vi "NewLINE.vi"() -> ()   [LabVIEW 2010]
uses:
  <vilib>/express/express arith-compare/Formula/XNode/ExpressFormulaBlockNode.xnode
panel:
  out "Numeric":u16
  in  "Array":dbl[](array[numeric])=[37.0]
  in  "Current (mA)":dbl
  in  "Motor GPIB":u8=6
  in  "y-dist":i32
  in  "speed":u16
  in  "x-dist":i32
  out "Dummy":string
  in  "Laser GPIB":u8=10 max=100
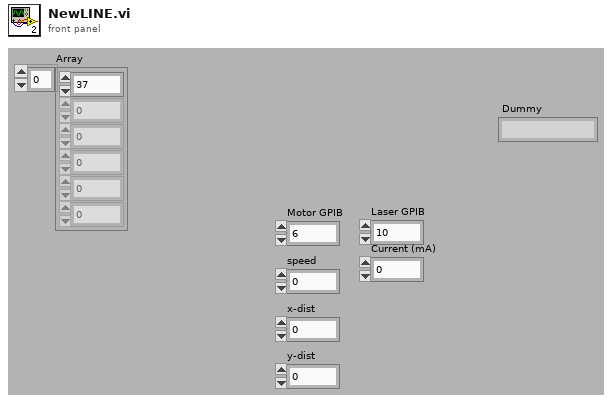
[diagram p1: front panel]
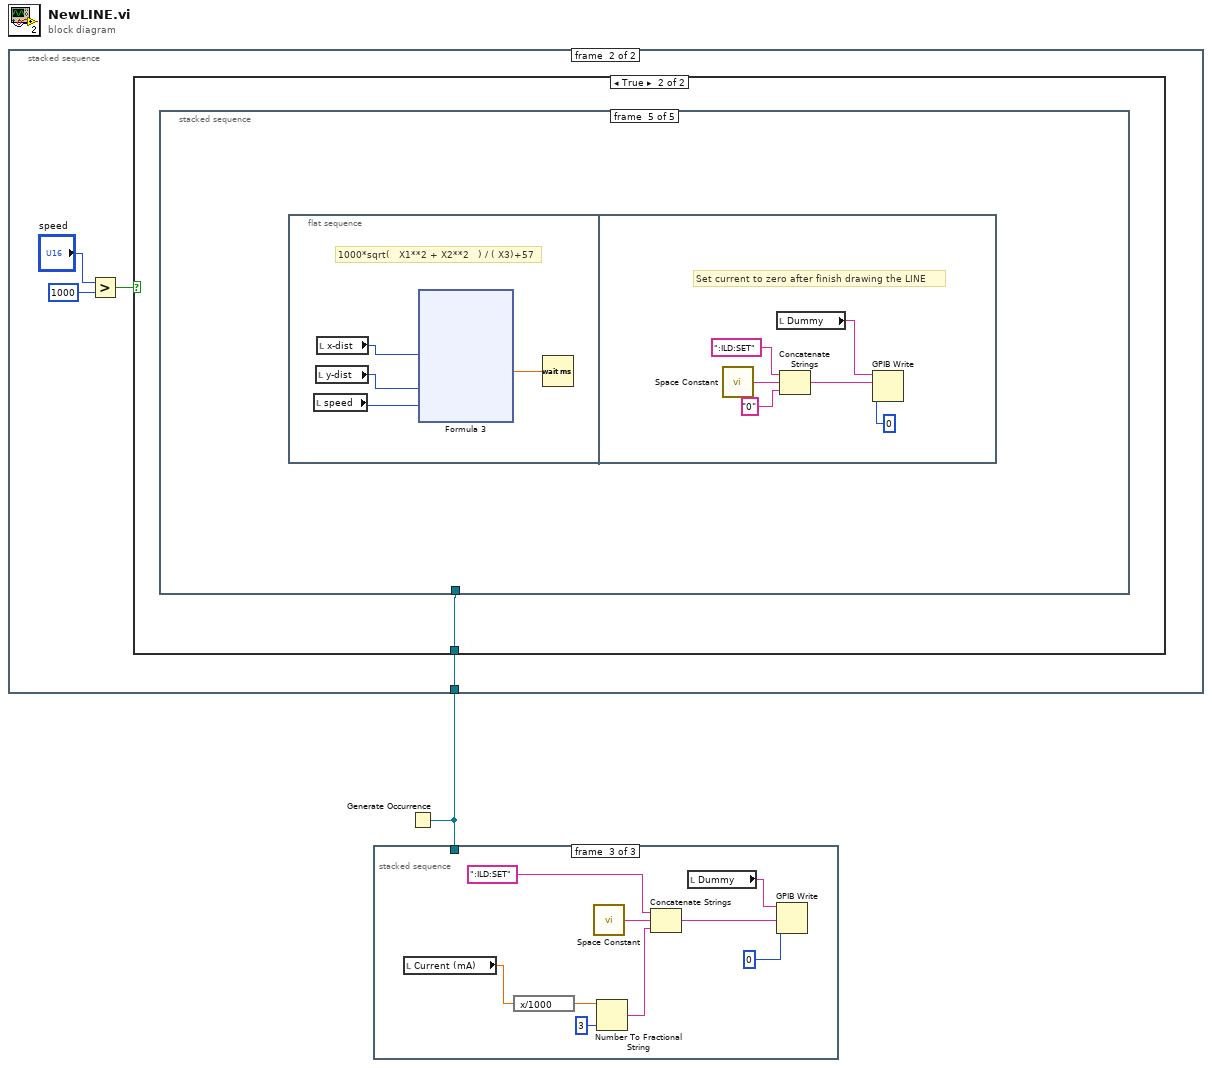
[diagram p0: block diagram]
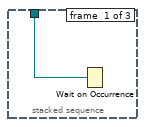
[diagram p2: hidden frame]
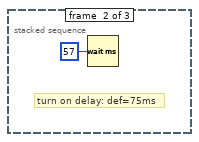
[diagram p3: hidden frame]
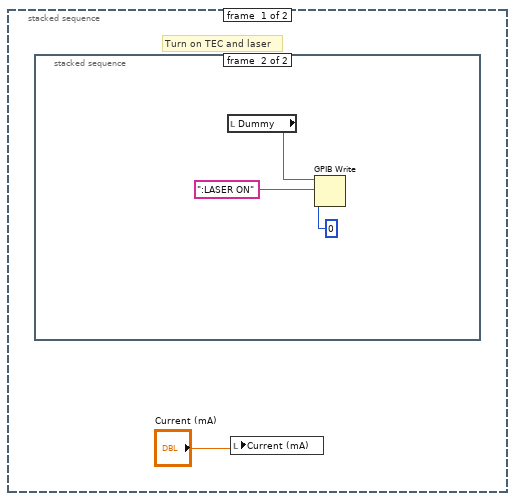
[diagram p4: hidden frame]
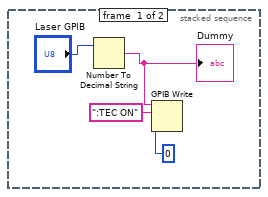
[diagram p5: hidden frame]
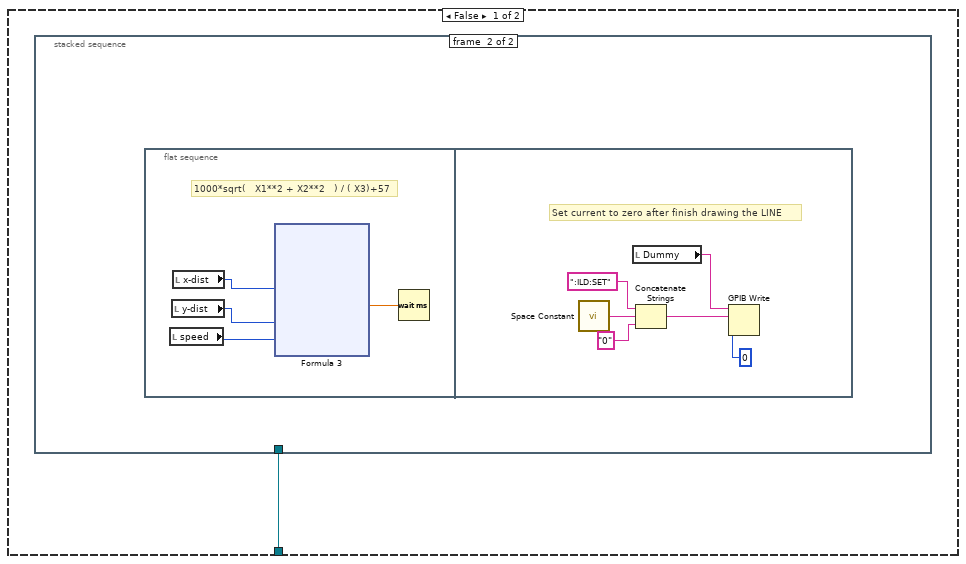
[diagram p6: hidden frame]
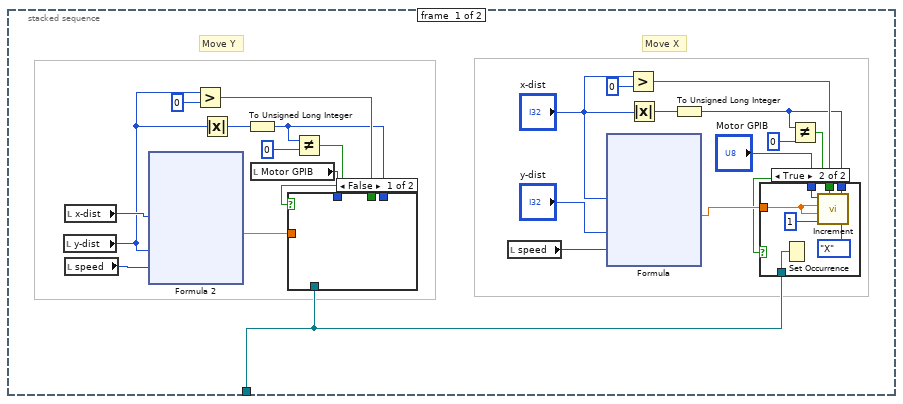
[diagram p7: hidden frame]
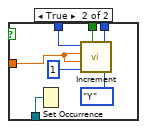
[diagram p9: hidden frame]
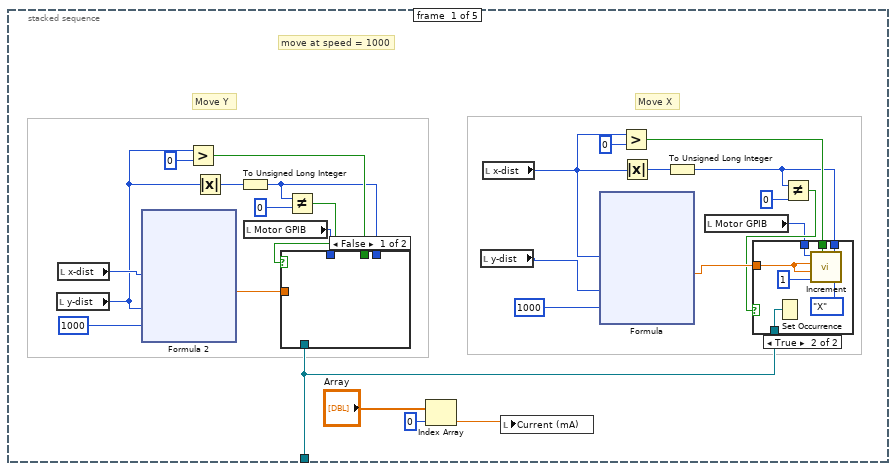
[diagram p10: hidden frame]
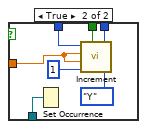
[diagram p12: hidden frame]
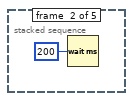
[diagram p13: hidden frame]
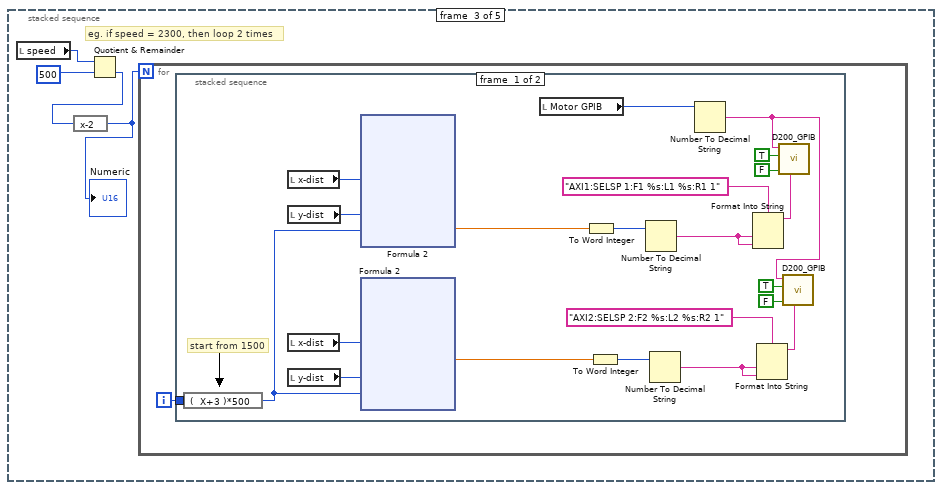
[diagram p14: hidden frame]
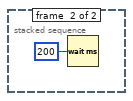
[diagram p15: hidden frame]
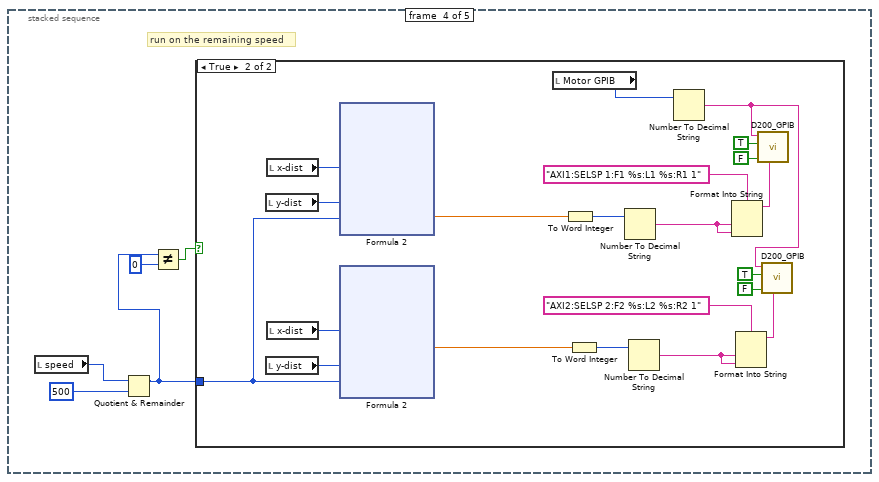
[diagram p16: hidden frame]
diagram:
  n1 = Generate Occurrence() -> (w1:refnum<k4>)
  n2 = stacked-sequence {
    tunnel: w1 -> [_ w11]
    frame #0 {
      # "Turn on TEC and laser"
      n3 = stacked-sequence {
        frame #0 {
          n4 = Number To Decimal String(number="Laser GPIB") -> (decimal integer string=w4:string)  [unwired: 1 in]
          "Dummy" <- w4
          n5 = GPIB Write(0:w4, 1:":TEC ON" ("data"), 2:i16 0 ("mode (0)")) -> ()  [unwired: 2 in, 2 out]
        }
        frame #1 {
          n6 = local read "Dummy"() -> (w8:string)
          n7 = GPIB Write(0:w8, 1:":LASER ON" ("data"), 2:i16 0 ("mode (0)")) -> ()  [unwired: 2 in, 2 out]
        }
      }
      n8 = local write "Current (mA)"("Current (mA)") -> ()
    }
    frame #1 {
      n9 = Greater?(x="speed", y=u16 1000) -> (0:w10:bool)
      n10 = case shown="True" w10 {
        tunnel: w11 -> [w14 w98]
        frame False {
          n11 = stacked-sequence {
            tunnel: w14 -> [w15 _]
            frame #0 {
              # "Move X"
              # "Move Y"
              n12 = local read "y-dist"() -> (w31:i32)
              n13 = local read "x-dist"() -> (w33:i32)
              n14 = local read "speed"() -> (w37:u16)
              n15 = xnode "Formula 2"("X1"=w33, "X2"=w31, "X3"=w37) -> ("Result"=w24:dbl)  [unwired: 1 in, 1 out]
              n16 = Greater?(x=w31, y=0) -> (0:w34:bool)
              n17 = Absolute Value(x=w31) -> (abs(x)=w32:i32)
              n18 = To Unsigned Long Integer(number=w32) -> (unsigned 32bit integer=w22:u32)
              n19 = local read "Motor GPIB"() -> (w36:u8)
              n20 = Not Equal?(x=w22, y=u32 0) -> (x != y?=w20:bool)
              n21 = case shown="False" w20 {
                tunnel: w36 -> [_ w49]
                tunnel: w34 -> [_ w48]
                tunnel: w22 -> [_ w47]
                tunnel: w24 -> [_ w46]
                tunnel: w15 -> [_ w45]
                frame False {
                }
                frame True {
                  n22 = Set Occurrence(w45) -> ()
                  n23 = call "Increment.vi"("GPIB_Addr"=w49, "F Speed"=w46, "L Speed"=w46, "Rate"=u16 1, "CCW 3"=w48, "Distance"=w47, "Axis"=enum16{"X", "Y", "Z", "U", "V", "W"}."Y") -> ()
                }
              }
              n24 = local read "speed"() -> (w16:u16)
              n25 = xnode "Formula"("X1"="x-dist", "X2"="y-dist", "X3"=w16) -> ("Result"=w23:dbl)  [unwired: 1 in, 1 out]
              n26 = Greater?(x="x-dist", y=0) -> (0:w28:bool)
              n27 = Absolute Value(x="x-dist") -> (abs(x)=w25:i32)
              n28 = To Unsigned Long Integer(number=w25) -> (unsigned 32bit integer=w19:u32)
              n29 = Not Equal?(x=w19, y=u32 0) -> (x != y?=w17:bool)
              n30 = case shown="True" w17 {
                tunnel: "Motor GPIB" -> [_ w44]
                tunnel: w28 -> [_ w41]
                tunnel: w19 -> [_ w40]
                tunnel: w23 -> [_ w39]
                tunnel: w15 -> [_ w38]
                frame False {
                }
                frame True {
                  n31 = Set Occurrence(w38) -> ()
                  n32 = call "Increment.vi"("GPIB_Addr"=w44, "F Speed"=w39, "L Speed"=w39, "Rate"=u16 1, "CCW 3"=w41, "Distance"=w40, "Axis"=enum16{"X", "Y", "Z", "U", "V", "W"}."X") -> ()
                }
              }
            }
            frame #1 {
              n33 = flat-sequence {
                frame #0 {
                  # "1000*sqrt(   X1**2 + X2**2   ) / ( X3)+57"
                  n34 = local read "speed"() -> (w76:u16)
                  n35 = local read "y-dist"() -> (w77:i32)
                  n36 = local read "x-dist"() -> (w78:i32)
                  n37 = xnode "Formula 3"("X1"=w78, "X2"=w77, "X3"=w76) -> ("Result"=w79:dbl)  [unwired: 1 in, 1 out]
                  n38 = Wait (ms)(milliseconds to wait=w79) -> ()  [unwired: 1 out]
                }
                frame #1 {
                  # "Set current to zero after finish drawing the LINE"
                  n39 = call <vilib>:"Space Constant.vi"() -> ("String"=w95:string)
                  n40 = local read "Dummy"() -> (w92:string)
                  n41 = Concatenate Strings(":ILD:SET", w95, "0" ("string")) -> (w94:string)
                  n42 = GPIB Write(0:w92, 1:w94, 2:i16 0 ("mode (0)")) -> ()  [unwired: 2 in, 2 out]
                }
              }
            }
          }
        }
        frame True {
          n43 = stacked-sequence {
            tunnel: w98 -> [w107 _ _ _ _]
            frame #0 {
              # "move at speed = 1000"
              # "Move X"
              # "Move Y"
              n44 = local read "y-dist"() -> (w119:i32)
              n45 = local read "x-dist"() -> (w121:i32)
              n46 = xnode "Formula 2"("X1"=w121, "X2"=w119, "X3"=u16 1000) -> ("Result"=w115:dbl)  [unwired: 1 in, 1 out]
              n47 = Greater?(x=w119, y=0) -> (0:w122:bool)
              n48 = Absolute Value(x=w119) -> (abs(x)=w120:i32)
              n49 = To Unsigned Long Integer(number=w120) -> (unsigned 32bit integer=w113:u32)
              n50 = local read "Motor GPIB"() -> (w124:u8)
              n51 = Not Equal?(x=w113, y=u32 0) -> (x != y?=w111:bool)
              n52 = case shown="False" w111 {
                tunnel: w124 -> [_ w136]
                tunnel: w122 -> [_ w135]
                tunnel: w113 -> [_ w134]
                tunnel: w115 -> [_ w133]
                tunnel: w107 -> [_ w132]
                frame False {
                }
                frame True {
                  n53 = Set Occurrence(w132) -> ()
                  n54 = call "Increment.vi"("GPIB_Addr"=w136, "F Speed"=w133, "L Speed"=w133, "Rate"=u16 1, "CCW 3"=w135, "Distance"=w134, "Axis"=enum16{"X", "Y", "Z", "U", "V", "W"}."Y") -> ()
                }
              }
              n55 = Index Array(array="Array", index=0) -> (element=w101:dbl)
              n56 = local read "y-dist"() -> (w103:i32)
              n57 = local read "x-dist"() -> (w104:i32)
              n58 = local write "Current (mA)"(w101) -> ()
              n59 = xnode "Formula"("X1"=w104, "X2"=w103, "X3"=u16 1000) -> ("Result"=w114:dbl)  [unwired: 1 in, 1 out]
              n60 = Greater?(x=w104, y=0) -> (0:w117:bool)
              n61 = Absolute Value(x=w104) -> (abs(x)=w116:i32)
              n62 = To Unsigned Long Integer(number=w116) -> (unsigned 32bit integer=w110:u32)
              n63 = local read "Motor GPIB"() -> (w102:u8)
              n64 = Not Equal?(x=w110, y=u32 0) -> (x != y?=w108:bool)
              n65 = case shown="True" w108 {
                tunnel: w102 -> [_ w131]
                tunnel: w117 -> [_ w128]
                tunnel: w110 -> [_ w127]
                tunnel: w114 -> [_ w126]
                tunnel: w107 -> [_ w125]
                frame False {
                }
                frame True {
                  n66 = Set Occurrence(w125) -> ()
                  n67 = call "Increment.vi"("GPIB_Addr"=w131, "F Speed"=w126, "L Speed"=w126, "Rate"=u16 1, "CCW 3"=w128, "Distance"=w127, "Axis"=enum16{"X", "Y", "Z", "U", "V", "W"}."X") -> ()
                }
              }
            }
            frame #1 {
              n68 = Wait (ms)(milliseconds to wait=u32 200) -> ()  [unwired: 1 out]
            }
            frame #2 {
              # "eg. if speed = 2300, then loop 2 times"
              n69 = local read "speed"() -> (w167:u16)
              n70 = Quotient & Remainder(x=w167, y=u16 500) -> (floor(x/y)=w165:u16)  [unwired: 1 out]
              n71 = expression code="x-2"(w165) -> (w164:u16)
              "Numeric" <- w164
              n72 = for {
                N: w164 -> [_]
                i -> [w168]
                n73 = stacked-sequence {
                  tunnel: w168 -> [w190 _]
                  frame #0 {
                    # "start from 1500"
                    n74 = expression code="(  X+3 )*500"(w190) -> (w178:i32)
                    n75 = local read "x-dist"() -> (w182:i32)
                    n76 = local read "y-dist"() -> (w181:i32)
                    n77 = local read "x-dist"() -> (w179:i32)
                    n78 = local read "y-dist"() -> (w180:i32)
                    n79 = xnode "Formula 2"("X1"=w182, "X2"=w181, "X3"=w178) -> ("Result"=w183:dbl)  [unwired: 1 in, 1 out]
                    n80 = xnode "Formula 2"("X1"=w179, "X2"=w180, "X3"=w178) -> ("Result"=w171:dbl)  [unwired: 1 in, 1 out]
                    n81 = local read "Motor GPIB"() -> (w169:u8)
                    n82 = To Word Integer(number=w183) -> (16bit integer=w184:i16)
                    n83 = To Word Integer(number=w171) -> (16bit integer=w177:i16)
                    n84 = Number To Decimal String(number=w184) -> (decimal integer string=w188:string)  [unwired: 1 in]
                    n85 = Number To Decimal String(number=w177) -> (decimal integer string=w173:string)  [unwired: 1 in]
                    n86 = Number To Decimal String(number=w169) -> (decimal integer string=w170:string)  [unwired: 1 in]
                    n87 = Format Into String(format string="AXI1:SELSP 1:F1 %s:L1 %s:R1 1", w188, w188) -> (resulting string=w189:string)  [unwired: 2 in, 1 out]
                    n88 = Format Into String(format string="AXI2:SELSP 2:F2 %s:L2 %s:R2 1", w173, w173) -> (resulting string=w172:string)  [unwired: 2 in, 1 out]
                    n89 = call "D200_GPIB.vi"("GPIB\nAddress"=w170, "Write"=TRUE, "Read"=FALSE, "Characters to Write"=w189) -> ()  [unwired: 1 in, 3 out]
                    n90 = call "D200_GPIB.vi"("GPIB\nAddress"=w170, "Write"=TRUE, "Read"=FALSE, "Characters to Write"=w172) -> ()  [unwired: 1 in, 3 out]
                  }
                  frame #1 {
                    n91 = Wait (ms)(milliseconds to wait=u32 200) -> ()  [unwired: 1 out]
                  }
                }
              }
            }
            frame #3 {
              # "run on the remaining speed"
              n92 = local read "speed"() -> (w219:u16)
              n93 = Quotient & Remainder(x=w219, y=u16 500) -> (x-y*floor(x/y)=w218:u16)  [unwired: 1 out]
              n94 = Not Equal?(x=w218, y=u16 0) -> (x != y?=w216:bool)
              n95 = case shown="True" w216 {
                tunnel: w218 -> [_ w221]
                frame False {
                }
                frame True {
                  n96 = local read "y-dist"() -> (w232:i32)
                  n97 = local read "y-dist"() -> (w231:i32)
                  n98 = local read "x-dist"() -> (w233:i32)
                  n99 = local read "x-dist"() -> (w230:i32)
                  n100 = xnode "Formula 2"("X1"=w233, "X2"=w232, "X3"=w221) -> ("Result"=w234:dbl)  [unwired: 1 in, 1 out]
                  n101 = xnode "Formula 2"("X1"=w230, "X2"=w231, "X3"=w221) -> ("Result"=w223:dbl)  [unwired: 1 in, 1 out]
                  n102 = local read "Motor GPIB"() -> (w241:u8)
                  n103 = To Word Integer(number=w234) -> (16bit integer=w235:i16)
                  n104 = To Word Integer(number=w223) -> (16bit integer=w229:i16)
                  n105 = Number To Decimal String(number=w235) -> (decimal integer string=w239:string)  [unwired: 1 in]
                  n106 = Number To Decimal String(number=w229) -> (decimal integer string=w225:string)  [unwired: 1 in]
                  n107 = Number To Decimal String(number=w241) -> (decimal integer string=w222:string)  [unwired: 1 in]
                  n108 = Format Into String(format string="AXI1:SELSP 1:F1 %s:L1 %s:R1 1", w239, w239) -> (resulting string=w240:string)  [unwired: 2 in, 1 out]
                  n109 = Format Into String(format string="AXI2:SELSP 2:F2 %s:L2 %s:R2 1", w225, w225) -> (resulting string=w224:string)  [unwired: 2 in, 1 out]
                  n110 = call "D200_GPIB.vi"("GPIB\nAddress"=w222, "Write"=TRUE, "Read"=FALSE, "Characters to Write"=w240) -> ()  [unwired: 1 in, 3 out]
                  n111 = call "D200_GPIB.vi"("GPIB\nAddress"=w222, "Write"=TRUE, "Read"=FALSE, "Characters to Write"=w224) -> ()  [unwired: 1 in, 3 out]
                }
              }
            }
            frame #4 {
              n112 = flat-sequence {
                frame #0 {
                  # "1000*sqrt(   X1**2 + X2**2   ) / ( X3)+57"
                  n113 = local read "speed"() -> (w266:u16)
                  n114 = local read "y-dist"() -> (w267:i32)
                  n115 = local read "x-dist"() -> (w268:i32)
                  n116 = xnode "Formula 3"("X1"=w268, "X2"=w267, "X3"=w266) -> ("Result"=w269:dbl)  [unwired: 1 in, 1 out]
                  n117 = Wait (ms)(milliseconds to wait=w269) -> ()  [unwired: 1 out]
                }
                frame #1 {
                  # "Set current to zero after finish drawing the LINE"
                  n118 = call <vilib>:"Space Constant.vi"() -> ("String"=w285:string)
                  n119 = local read "Dummy"() -> (w282:string)
                  n120 = Concatenate Strings(":ILD:SET", w285, "0" ("string")) -> (w284:string)
                  n121 = GPIB Write(0:w282, 1:w284, 2:i16 0 ("mode (0)")) -> ()  [unwired: 2 in, 2 out]
                }
              }
            }
          }
        }
      }
    }
  }
  n122 = stacked-sequence {
    tunnel: w1 -> [w288 _ _]
    frame #0 {
      n123 = Wait on Occurrence(2:w288) -> ()  [unwired: 2 in, 1 out]
    }
    frame #1 {
      # "turn on delay: def=75ms"
      n124 = Wait (ms)(milliseconds to wait=u32 57) -> ()  [unwired: 1 out]
    }
    frame #2 {
      n125 = local read "Current (mA)"() -> (w296:dbl)
      n126 = expression code="x/1000"(w296) -> (w295:dbl)
      n127 = call <vilib>:"Space Constant.vi"() -> ("String"=w291:string)
      n128 = Number To Fractional String(number=w295, precision (6)=i16 3) -> (F-format string=w293:string)  [unwired: 2 in]
      n129 = Concatenate Strings(":ILD:SET", w291, w293) -> (w290:string)
      n130 = local read "Dummy"() -> (w298:string)
      n131 = GPIB Write(0:w298, 1:w290, 2:i16 0 ("mode (0)")) -> ()  [unwired: 2 in, 2 out]
    }
  }
